vi "LOAD SELECTION MAIN CODE.vi"(8 "error in (no error)":errorcluster, 11 "main ref":T1) -> (0 "error out":errorcluster)   [LabVIEW 2025]
uses:
  controls/LAB-IQ UI Data.ctl
  <vilib>/addons/control/pid/pid.llb/PID Output Rate Limiter (DBL).vi
  <vilib>/addons/control/pid/NI_PID_pid.lvlib
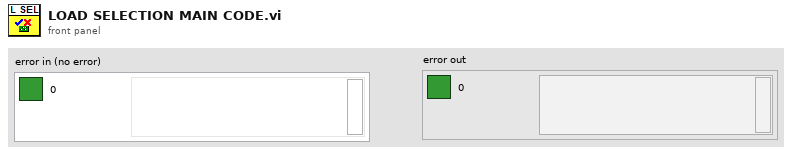
[diagram p1: front panel]
types:
  T1 = typedef "LAB-IQ UI Data.ctl" = cluster{"Main Home Screen":cluster{"GUI":refnum<vi>, "Platform Settings":refnum<vi>, "Configure":refnum<vi>, "Home":refnum<vi>, "EXIT":refnum<vi>, "service 2":refnum<vi>, "MainPage":refnum<vi>, "Analysis":refnum<vi>}, "Platform Settings":cluster{"mm/s  Surge":refnum<vi>, "Update Surge Speed":refnum<vi>, "Drive Error":refnum<vi>, "Disable Axis Jog Soft Limits":refnum<vi>, "mm/s  Sway":refnum<vi>, "Sway and Surge COM Status":refnum<vi>, "Heave COM Status":refnum<vi>, "Enable Platform":refnum<vi>, "Surge Forward Main":refnum<vi>, "Sway Right Main":refnum<vi>, "Sway Left Main":refnum<vi>, "Heave Down Main":refnum<vi>, "Heave Up main":refnum<vi>, "Update Sway Speed":refnum<vi>, "Update Heave Speed":refnum<vi>, "mm/s Heave":refnum<vi>, "mm/sec":refnum<vi>, "mm":refnum<vi>, "Surge Backward Main":refnum<vi>}, "Analysis Screen":cluster{"Analysis Home":refnum<vi>, "Surface Analysis":refnum<vi>, "Imaging":refnum<vi>, "Image Analysis":refnum<vi>, "Post Analysis":refnum<vi>}, "Config Screen":cluster{"Select Load Head":refnum<vi>, "Notes :":refnum<vi>, "FILE":refnum<vi>, "Sample ID :":refnum<vi>, "Operator ID :":refnum<vi>, "Operator Name :":refnum<vi>, "Auto":refnum<vi>}, "Motion Module":cluster{"zNL":refnum<vi>, "NL disp":refnum<vi>, "Rotary Tab":refnum<vi>, "Motion Direction:  3":refnum<vi>, "E.Velocity 2":refnum<vi>, "e.v/ssr 2":refnum<vi>, "Enter Fixed E.Velocity 2":refnum<vi>, "Enter Final SRR 2":refnum<vi>, "Enter initial SRR 2":refnum<vi>, "Enter Fixed SRR 2":refnum<vi>, "Enter the Final E.Velocity (m/s) 2":refnum<vi>, "Enter initial E.Velocity (m/s) 2":refnum<vi>, "Final Speed (RPM) 3":refnum<vi>, "Initial Speed (RPM) 2":refnum<vi>, "Enter the Final Velocity (m/s) 3":refnum<vi>, "Enter initial Velocity (m/s)  3":refnum<vi>, "Ramp Up 2":refnum<vi>, "TEST SELECTION":refnum<vi>, "SPEED SELECTION : ":refnum<vi>, "Angular Oscillation Set":refnum<vi>, "Traction":refnum<vi>, "Step Speed":refnum<vi>, "StepTable For Load-Speed":refnum<vi>, "StepTable For Speed":refnum<vi>, "Surge Forward MM":refnum<vi>, "Surge Backward MM":refnum<vi>, "M3 Image":refnum<vi>, "String 39":refnum<vi>, "Sway Left MM":refnum<vi>, "Sway Right MM":refnum<vi>, "Disable Axis Jog Soft Limits":refnum<vi>, "mm":refnum<vi>, "Heave Down MM":refnum<vi>, "Heave Up MM":refnum<vi>, "Wear Track Diameter (mm)":refnum<vi>, "Set WTD":refnum<vi>, "HomeScratch":refnum<vi>, "HomeRot":refnum<vi>, "PlaceModule":refnum<vi>, "Enter the Angle (Deg)":refnum<vi>, "Enter the Frequency (Hz)":refnum<vi>, "Motion Mode:":refnum<vi>, "LR Sway":refnum<vi>, "Rot Hor":refnum<vi>, "Scratch":refnum<vi>, "LR Cam":refnum<vi>, "MMBack":refnum<vi>, "MMNext":refnum<vi>, "Rot Ver":refnum<vi>, "Rotary Module Selection":refnum<vi>, "calculate rotary":refnum<vi>, "SPEED SELECTION : rotary":refnum<vi>, "Import 2":refnum<vi>, "Save 2":refnum<vi>, "File Path :  2":refnum<vi>, "String 45":refnum<vi>, "StepTable For Speed 3":refnum<vi>, "Enter the Speed(mm/sec)":refnum<vi>, "Enter the Speed(RPM)":refnum<vi>, "Enter Scratch Speed (mm/s):":refnum<vi>, "SwaySpeed Set":refnum<vi>, "Scartch Offset":refnum<vi>, "Motion type:":refnum<vi>, "HomeScratch 2":refnum<vi>, "Enter Scratch length (mm):":refnum<vi>, "Wear Track Diameter":refnum<vi>, "Rotary Speed Exced":refnum<vi>, "Scratch Mode":refnum<vi>, "No of Scratch":refnum<vi>}, "Environmental control":cluster{"Humidity  Status  3":refnum<vi>, "Low Temp  Status  2":refnum<vi>, "TK4 status 2":refnum<vi>, "Stage Temperature":refnum<vi>, "Sample Temperature":refnum<vi>, "Humidity (Amb)":refnum<vi>, "Clear List":refnum<vi>, "Add to list":refnum<vi>, "Wear":refnum<vi>, "Vibration":refnum<vi>, "Humidity (Chamber)":refnum<vi>, "Temperature (Chamber)":refnum<vi>, "ECR ":refnum<vi>, "Temperature (Amb)":refnum<vi>, "Microphone":refnum<vi>, "Acoustic Emission 3":refnum<vi>, "SNext":refnum<vi>, "APBack":refnum<vi>, "Enter the Temperature (°C):":refnum<vi>, "Enter the Stage \nTemperature (°C):":refnum<vi>, "Enter the Humidity (%Rh):":refnum<vi>, "Low Temp":refnum<vi>, "High Temp":refnum<vi>, "Humidity":refnum<vi>, "Sensors Picked":refnum<vi>}, "About Screen":cluster{"Password":refnum<vi>, "Home Service":refnum<vi>, "Advanced Setting":refnum<vi>, "About Tab":refnum<vi>, "ECR Port:":refnum<vi>, "Ramp Port:":refnum<vi>, "Installation/Replacement completed":refnum<vi>, "Loahead":refnum<vi>, "Heave and Surge COM Port:":refnum<vi>, "Sway COM Port:":refnum<vi>, "Temp Modbus:":refnum<vi>, "Humidity Port:":refnum<vi>, "Edit Gain Constants":refnum<vi>, "Save Gain Constants":refnum<vi>}, "Main Screen":cluster{"Main Screen Tab":refnum<vi>, "Angle and Frequency":refnum<vi>, "Stroke (mm)":refnum<vi>, "Angle (Deg)":refnum<vi>, "Main Speed Tab":refnum<vi>, "MTM MOTOR DISPLAY":refnum<vi>, "Disc Speed (m/sec)":refnum<vi>, "Ball Speed (m/sec)":refnum<vi>, "Disc Speed (RPM)":refnum<vi>, "Ball Speed (RPM)":refnum<vi>, "SPEED TAB":refnum<vi>, "Speed (m/sec)":refnum<vi>, "Set Speed (m/sec)":refnum<vi>, "Speed (RPM)":refnum<vi>, "Set Speed":refnum<vi>, "Time Tab":refnum<vi>, "Time ( HH:MM:SS ) 2":refnum<vi>, "Test Duration":refnum<vi>, "Test Duration 4":refnum<vi>, "TEST CYCLE":refnum<vi>, "TOTAL CYCLES":refnum<vi>, "Set Load (N)":refnum<vi>, "Temp Tabs":refnum<vi>, "Heater":refnum<vi>, "TK4 status":refnum<vi>, "ChamberTemp":refnum<vi>, "SetTmp":refnum<vi>, "Controller  Status":refnum<vi>, "ChamberTemp 2":refnum<vi>, "SetTmp 2":refnum<vi>, "Controller  Status 2":refnum<vi>, "ChamberTemp 3":refnum<vi>, "SetTmp 3":refnum<vi>, "Cooling":refnum<vi>, "Load Communication":refnum<vi>, "Ambient \nTemperature":refnum<vi>, "HumCOMStatus":refnum<vi>, "Ambient\n Humidity":refnum<vi>, "Freq (Hz)":refnum<vi>, "Load En":refnum<vi>, "NLt":refnum<vi>, "zNL 2":refnum<vi>, "Humidity On":refnum<vi>, "humidity disp":refnum<vi>, "Set Humidity":refnum<vi>, "NL disp 2":refnum<vi>, "Humidity On 2":refnum<vi>, "humidity disp 2":refnum<vi>, "Set Humidity 2":refnum<vi>, "NL disp 3":refnum<vi>, "AppLoadSeq scratch":refnum<vi>, "Stop Scratch":refnum<vi>, "ClrLog":refnum<vi>, "Trip Log":refnum<vi>, "STOP":refnum<vi>, "Start Test":refnum<vi>, "Test status":refnum<vi>, "AR Led":refnum<vi>, "Data":refnum<vi>, "Health":refnum<vi>, "Sway COM Status":refnum<vi>, "Heave COM Status":refnum<vi>, "Grp Tab":refnum<vi>, "Sub Graph":refnum<vi>, "SD (mm)":refnum<vi>, "Siliding distance Reset Graph":refnum<vi>, "SDGp":refnum<vi>, "Humidity Reset Graph":refnum<vi>, "HumrGp":refnum<vi>, "Acoustic Emission (mV)":refnum<vi>, "Aqucostic Reset Graph":refnum<vi>, "gACQUOS":refnum<vi>, "ECR RESET":refnum<vi>, "ECR":refnum<vi>, "Temperature Reset":refnum<vi>, "Acoustic Emission (mV) 2":refnum<vi>, "Aqucostic Reset Graph 2":refnum<vi>, "gACQUOS 2":refnum<vi>, "ECR RESET 2":refnum<vi>, "ECR 2":refnum<vi>, "Temperature Reset 2":refnum<vi>, "Temperature (deg c)":refnum<vi>, "Speed Reset Graph":refnum<vi>, "Speed Tab":refnum<vi>, "MTM DISC  SPEED":refnum<vi>, "MTM BALL SPEED":refnum<vi>, "speed mm/sec":refnum<vi>, "Hymidity":refnum<vi>, "Humidity Disable trip":refnum<vi>, "CoF Trip  2":refnum<vi>, "Depth Trip":refnum<vi>, "Weart Deapth":refnum<vi>, "Depth Reset Graph":refnum<vi>, "Weart":refnum<vi>, "Depthz":refnum<vi>, "Depth (µm)":refnum<vi>, "WearGp":refnum<vi>, "NL Trip 2":refnum<vi>, "Load pid":refnum<vi>, "Load Disable Trip":refnum<vi>, "Load Reset Graph":refnum<vi>, "NL Display 4":refnum<vi>, "Main Chart 3":refnum<vi>, "BACK":refnum<vi>, "Depth Trip 2":refnum<vi>, "COF TRIP ":refnum<vi>, "Friction Force (N)":refnum<vi>, "FF Reset Graph":refnum<vi>, "FF Disable Trip":refnum<vi>, "FF TRIP":refnum<vi>, "COF Disable Trip":refnum<vi>, "COF Reset Graph":refnum<vi>, "Start Test Temp":refnum<vi>, "zFF":refnum<vi>, "Friction Force (N) Graph":refnum<vi>, "Coefficient of Friction":refnum<vi>, "Scratch Start Test":refnum<vi>, "FF Tab":refnum<vi>, "Cyclic Friction Force (N)":refnum<vi>, "CZ FF":refnum<vi>, "Cyclic Friction Force (N) Graph":refnum<vi>, "Cyclic Coefficient of Friction":refnum<vi>, "Cyclic FF TRIP":refnum<vi>, "Cyclic FF Disable Trip":refnum<vi>, "cyclic COF Disable Trip":refnum<vi>, "cyclic COF TRIP":refnum<vi>, "cyclic COF Reset Graph":refnum<vi>, "Cyclic FF Reset Graph":refnum<vi>, "Test Trip":refnum<vi>, "Multi Scratch Pass":refnum<vi>}, "Loading":cluster{"Indentation":refnum<vi>, "Reference Sample":refnum<vi>, "Load Cell Communication Slide":refnum<vi>, "com 3":refnum<vi>, "com":refnum<vi>, "DecaForce COM Status":refnum<vi>, "Update":refnum<vi>, "Clear 3":refnum<vi>, "seq":refnum<vi>, "Stribeck table":refnum<vi>, "Stribeck Table  For loading":refnum<vi>, "Loading Mode":refnum<vi>, "Enter the Final Load (N)":refnum<vi>, "Enter the CoF Trip":refnum<vi>, "Enter the Friction Force Trip":refnum<vi>, "Enter the Normal load Trip":refnum<vi>, "Enter the Load  (N)":refnum<vi>, "KiloForce":refnum<vi>, "DecaForce ":refnum<vi>, "MicroForce":refnum<vi>, "LHBack":refnum<vi>, "LHNext":refnum<vi>, "Enter the Loading Rate (N/min)":refnum<vi>, "Message":refnum<vi>, "Warning 2":refnum<vi>, "SSP 0.75":refnum<vi>, "SSP 0.5":refnum<vi>, "SSP 0.3":refnum<vi>, "Warning":refnum<vi>, "gui GIF":refnum<vi>, "Communication is established":refnum<vi>, "AppLoad 4":refnum<vi>, "Multipoint":refnum<vi>, "Load Selection":refnum<vi>}, "PID":cluster{"Ramp MulFac":refnum<vi>, "pulses LoadDiffRamp(2..10)":refnum<vi>, "PulseControlRamp(diff<=3N)":refnum<vi>, "SetLoadDeadband(%) Load(0-10N)":refnum<vi>, "PID gains out delay (microForce)":refnum<vi>, "Ramp":refnum<vi>, "Gain 2":refnum<vi>, "pulses LoadDiff(2..10)":refnum<vi>, "pulses LoadDiff(11..50)":refnum<vi>, "PulseControl(diff<=3N)":refnum<vi>, "SetLoadDeadband(%)  2":refnum<vi>, "Dummy Run":refnum<vi>, "Vertical load (N)":refnum<vi>, "AutoTune":refnum<vi>, "Offset 3 ":refnum<vi>, "apply load":refnum<vi>, "Offset  3":refnum<vi>, "apply load 2":refnum<vi>, "Enter ByPass Load":refnum<vi>, "reinit 3":refnum<vi>, "output range delay":refnum<vi>, "PID gains out delay":refnum<vi>, "Bypass Load":refnum<vi>, "pulsesSent":refnum<vi>, "pulses ":refnum<vi>, "actpid":refnum<vi>, "gFF Rot":refnum<vi>, "pulses LoadDiff(21..1000)":refnum<vi>, "Delay":refnum<vi>, "deadband":refnum<vi>}, "Config Parameters":cluster{"Tab Control 3":refnum<vi>, "Tab Control 19":refnum<vi>, "SAMPLES":refnum<vi>, "Re-initilaize":refnum<vi>, "Filter ON/OFF":refnum<vi>, "TracHomeSurgeOffsetCounts 10MM":refnum<vi>, "TracHomeSwayOffsetCounts 10MM":refnum<vi>, "Acoustic Emission:":refnum<vi>, "Apply Filter (FF)":refnum<vi>, "Filter% 2":refnum<vi>, "Apply Filter (Load)":refnum<vi>, "Filter% ":refnum<vi>, "Sway distance (mm)":refnum<vi>, "Surge distance (mm)":refnum<vi>, "DataSavingLoopDelay(ms)":refnum<vi>, "SAVE 2":refnum<vi>, "Enter Distance":refnum<vi>, "Sway Counts:":refnum<vi>, "Distance (mm): 3":refnum<vi>, "Surge Counts:":refnum<vi>, "Distance (mm): 2":refnum<vi>, "Distance (mm):":refnum<vi>, "Heave Counts:":refnum<vi>, "LRMHomeSurgeOffsetCounts":refnum<vi>, "LRMHomeSwayOffsetCounts":refnum<vi>, "TracHomeSurgeOffsetCounts 20MM":refnum<vi>, "TracHomeSwayOffsetCounts 20MM":refnum<vi>, "RotHomeSwayOffsetCounts":refnum<vi>, "RotHomeSurgeOffsetCounts":refnum<vi>, "Heave distance":refnum<vi>, "Zmm":refnum<vi>, "Heave Pulses/mm":refnum<vi>, "Surge Pulses/mm":refnum<vi>, "Sway Pulses/mm":refnum<vi>, "Heave Pitch":refnum<vi>, "Surge Pitch":refnum<vi>, "Sway Pitch":refnum<vi>, "Heave PPR":refnum<vi>, "Surge PPR":refnum<vi>, "Sway PPR":refnum<vi>, "Tab Control 5":refnum<vi>, "Tab Control 14":refnum<vi>, "Tab Control 26":refnum<vi>, "AE":refnum<vi>, "Heave Loop Delay":refnum<vi>, "Heave PID Speed":refnum<vi>, "Surge Jog Speed":refnum<vi>, "Heave Jog Speed":refnum<vi>, "Sway Loop Delay":refnum<vi>, "Sway PID Speed":refnum<vi>, "Sway Jog Speed":refnum<vi>}, "Loading Com Port":cluster{"ClearAll":refnum<vi>, "Mz(Nm)":refnum<vi>, "My(Nm)":refnum<vi>, "Mx(Nm)":refnum<vi>, "Save Dwell":refnum<vi>, "Mx ":refnum<vi>, "My ":refnum<vi>, "Mz":refnum<vi>, "Fx(N)":refnum<vi>, "Fy(N)":refnum<vi>, "Fz(N)":refnum<vi>, "ZeroAll":refnum<vi>, "Acq Delay (ms)":refnum<vi>, "Burst Delay (ms)":refnum<vi>, "model":refnum<vi>, "SN":refnum<vi>, "FFx(N)":refnum<vi>, "Sensor IP":refnum<vi>, "Port":refnum<vi>, "FFy(N)":refnum<vi>, "Load(N)":refnum<vi>, "delete Handle":refnum<vi>, "Create Handle":refnum<vi>, "ft_data":refnum<vi>, "ft_range":refnum<vi>, "ft_data 2":refnum<vi>, "stop 6":refnum<vi>, "running_flag":refnum<vi>, "ft_udp_handle":refnum<vi>, "get-data-return":refnum<vi>, "get-range-return":refnum<vi>, "zero-return":refnum<vi>, "filter-return":refnum<vi>, "initial-return":refnum<vi>, "deleteHandle-result":refnum<vi>, "Load Cell Temp":refnum<vi>}, "Heave AND Surge":cluster{"SURGE POSE":refnum<vi>, "error out Read":refnum<vi>, "HEAVE POSE":refnum<vi>, "State":refnum<vi>, "Homed":refnum<vi>, "Sequence ID":refnum<vi>, "error out Write":refnum<vi>, "faultCode":refnum<vi>, "Ack ID":refnum<vi>, "SPEED":refnum<vi>, "Distance":refnum<vi>, "Mode Command":refnum<vi>, "Heave and Surge Read":refnum<vi>, "Read Heave Temp":refnum<vi>, "Spare 15":refnum<vi>, "Spare 14":refnum<vi>, "Spare 13":refnum<vi>, "Spare 12":refnum<vi>, "Spare 11":refnum<vi>, "Spare 10":refnum<vi>, "Spare 9":refnum<vi>, "Spare 8":refnum<vi>, "Spare 7":refnum<vi>, "Spare 6":refnum<vi>, "Spare 5":refnum<vi>, "Spare 4":refnum<vi>, "Spare 2":refnum<vi>, "Spare 1":refnum<vi>, "Node Id":refnum<vi>, "Spare 3":refnum<vi>, "SPARE 4":refnum<vi>, "SPARE 3":refnum<vi>, "SPARE 2":refnum<vi>, "SPARE 1":refnum<vi>, "fwMajor":refnum<vi>, "fwMinor":refnum<vi>, "Manual Write":refnum<vi>, "Heave and Surge Write":refnum<vi>}, "New PID LOGIC":cluster{"Fine Tune Zone":refnum<vi>, "PID SDelay":refnum<vi>, "Max_pos_limit":refnum<vi>, "Min_pos_limit":refnum<vi>, "i_limit":refnum<vi>, "pct_scale":refnum<vi>, "Deadband":refnum<vi>, "Kd":refnum<vi>, "Ki":refnum<vi>, "Kp":refnum<vi>, "Current Position":refnum<vi>, "Set Load":refnum<vi>, "Current Load":refnum<vi>, "Pulse delta":refnum<vi>, "Init Step":refnum<vi>, "Max Step Linit":refnum<vi>}, "SWAY ":cluster{"fwMajor":refnum<vi>, "Homed":refnum<vi>, "Rotary POSE":refnum<vi>, "State":refnum<vi>, "SWAY POSE":refnum<vi>, "Ack ID":refnum<vi>, "faultCode":refnum<vi>, "Node Id":refnum<vi>, "fwMinor":refnum<vi>, "Spare 6":refnum<vi>, "Spare 5":refnum<vi>, "Spare 4":refnum<vi>, "Spare 3":refnum<vi>, "Spare 2":refnum<vi>, "Spare 1":refnum<vi>, "Spare 7":refnum<vi>, "SPARE  5":refnum<vi>, "error out Write  SWAY ":refnum<vi>, "error out Read SWAY ":refnum<vi>, "Manual Write SWAY ":refnum<vi>, "SWAY WRITE":refnum<vi>, "SPARE  4":refnum<vi>, "SPARE  3":refnum<vi>, "SPARE 2":refnum<vi>, "SPARE 1":refnum<vi>, "Spare 15":refnum<vi>, "Spare 14":refnum<vi>, "Spare 13":refnum<vi>, "Spare 12":refnum<vi>, "Spare 11":refnum<vi>, "Spare 9":refnum<vi>, "Spare 8":refnum<vi>, "SPEED":refnum<vi>, "Distance":refnum<vi>, "Mode Command":refnum<vi>, "Sequence ID":refnum<vi>, "SWAY READ":refnum<vi>, "Spare 10":refnum<vi>, "Read SWAY Temp":refnum<vi>}, "Analysis Screen":cluster{"Analysis Home":refnum<vi>, "Refresh 2":refnum<vi>, "MEAN 4":refnum<vi>, "SD 4":refnum<vi>, "VARIANCE 4":refnum<vi>, "MEAN  3":refnum<vi>, "SD  3":refnum<vi>, "VARIANCE  3":refnum<vi>, "MEAN 2":refnum<vi>, "SD  2":refnum<vi>, "VARIANCE 2":refnum<vi>, "MEAN":refnum<vi>, "SD":refnum<vi>, "VARIANCE":refnum<vi>, "File 4 Discription":refnum<vi>, "OPEN 4":refnum<vi>, "File Name 4":refnum<vi>, "OPEN 3":refnum<vi>, "File 3 Discription":refnum<vi>, "File Name 3":refnum<vi>, "Y-AXIS":refnum<vi>, "X-AXIS":refnum<vi>, "XY Graph":refnum<vi>, "File Name 2":refnum<vi>, "File Name 1":refnum<vi>, "OPEN 2":refnum<vi>, "OPEN 1":refnum<vi>, "File 1 Discription ":refnum<vi>, "File 2 Discription":refnum<vi>}}
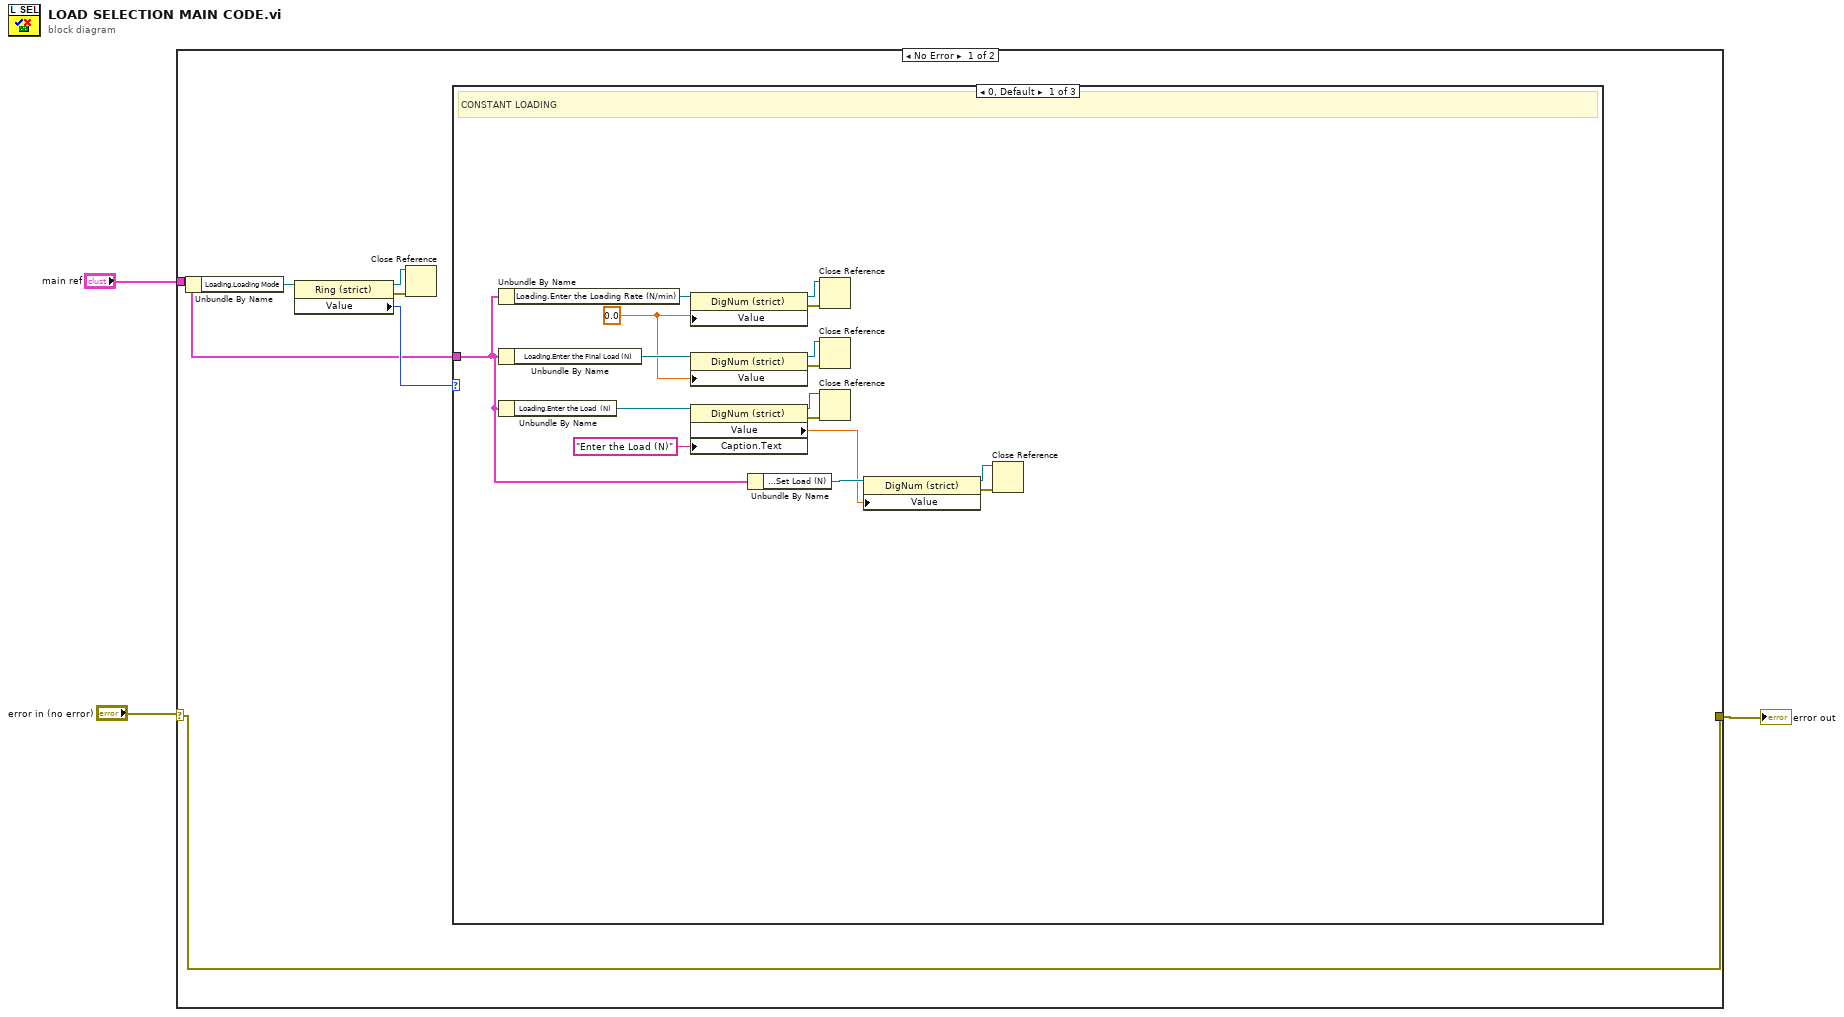
[diagram p0: block diagram]
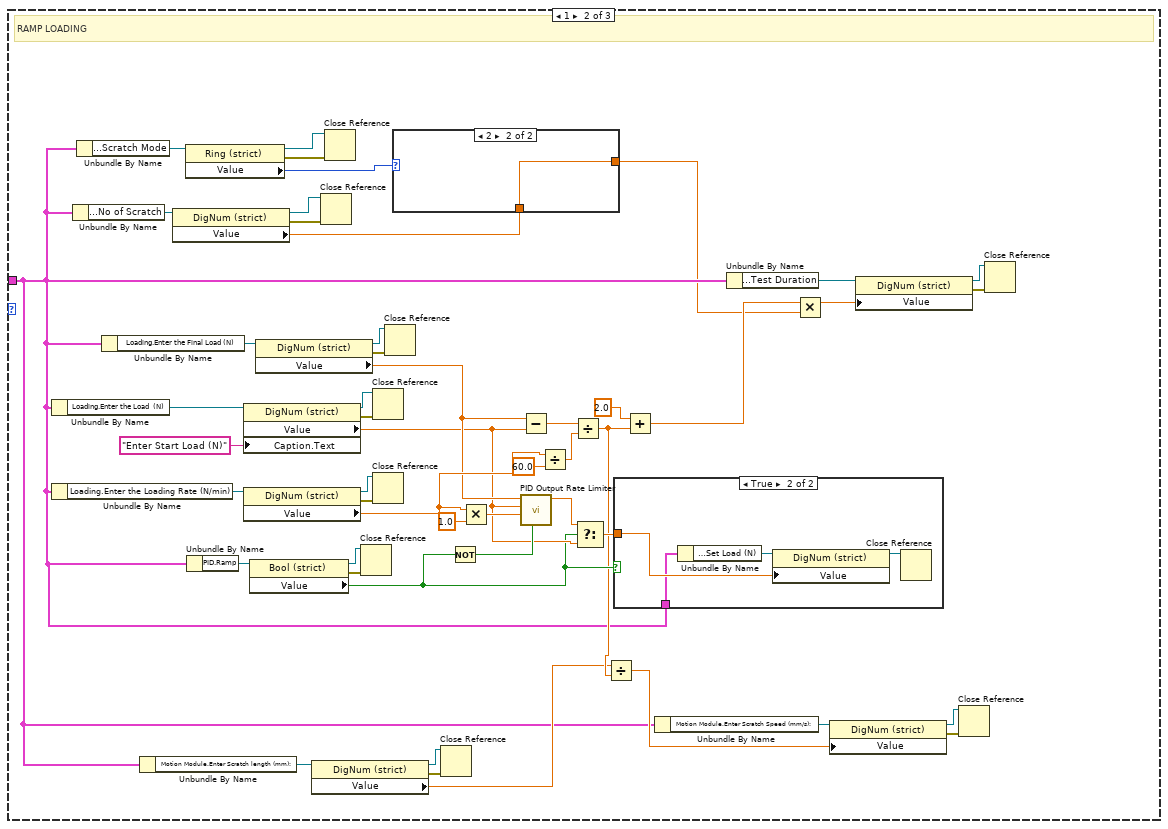
[diagram p2: hidden frame]
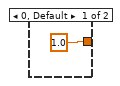
[diagram p3: hidden frame]
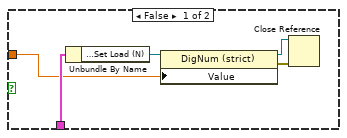
[diagram p4: hidden frame]
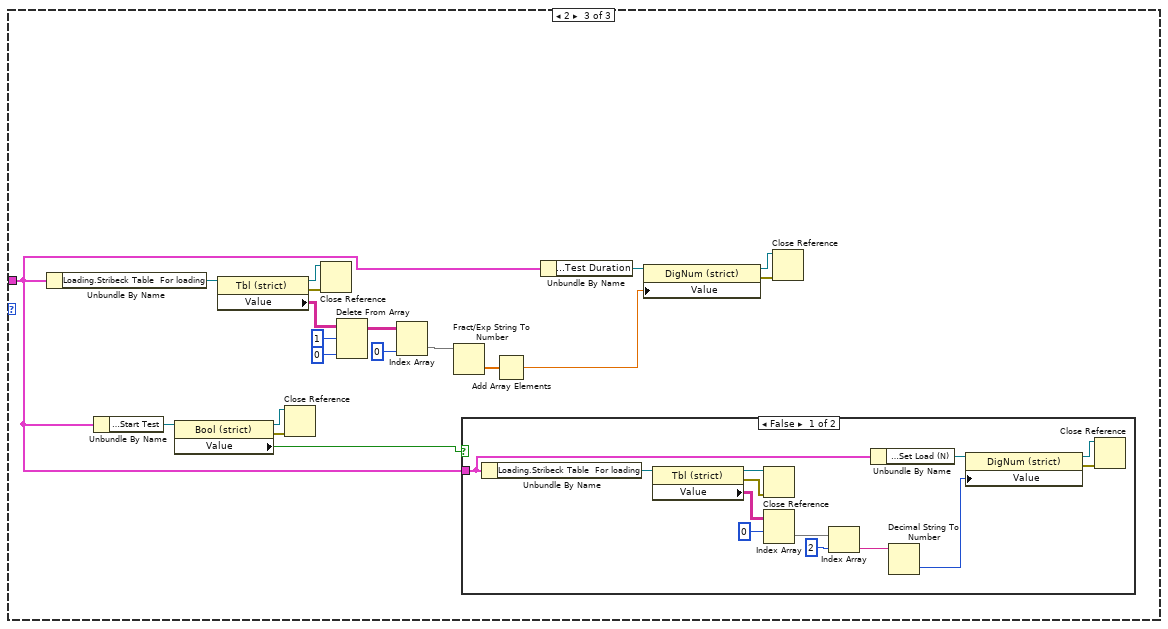
[diagram p5: hidden frame]
diagram:
  n1 = case shown="No Error" "error in (no error)" {
    selector: "error in (no error)" -> [w4 _]
    tunnel: "main ref" -> [w5 _]
    tunnel: [w4 _] -> w1
    frame No Error {
      n2 = Unbundle By Name(w5) -> ("Loading.Loading Mode"=w9:refnum<vi>)
      n3 = property class="Ring (strict)"(reference=w9) -> (reference out=w7:refnum<vi>, error out=w8:errorcluster, "Value"=w6:u16)  [unwired: 1 in]
      n4 = Close Reference(reference=w7, error in (no error)=w8) -> ()  [unwired: 1 out]
      n5 = case shown="0, Default" w6 {
        tunnel: w5 -> [w12 w28 w89]
        frame 0, Default {
          w16 = 0.0 ("Value")
          # "CONSTANT LOADING"
          n6 = Unbundle By Name(w12) -> ("Loading.Enter the Loading Rate (N/min)"=w19:refnum<vi>)
          n7 = Unbundle By Name(w12) -> ("Loading.Enter the Final Load (N)"=w23:refnum<vi>)
          n8 = Unbundle By Name(w12) -> ("Loading.Enter the Load  (N)"=w22:refnum<vi>)
          n9 = property class="DigNum (strict)"(reference=w19, "Value"=w16) -> (reference out=w17:refnum<vi>, error out=w18:errorcluster)  [unwired: 1 in]
          n10 = property class="DigNum (strict)"(reference=w23, "Value"=w16) -> (reference out=w25:refnum<vi>, error out=w24:errorcluster)  [unwired: 1 in]
          n11 = property class="DigNum (strict)"(reference=w22, "Caption.Text"="Enter the Load (N)") -> (reference out=w20:refnum<vi>, error out=w21:errorcluster, "Value"=w11:dbl)  [unwired: 1 in]
          n12 = Unbundle By Name(w12) -> ("Main Screen.Set Load (N)"=w13:refnum<vi>)
          n13 = Close Reference(reference=w17, error in (no error)=w18) -> ()  [unwired: 1 out]
          n14 = Close Reference(reference=w25, error in (no error)=w24) -> ()  [unwired: 1 out]
          n15 = Close Reference(reference=w20, error in (no error)=w21) -> ()  [unwired: 1 out]
          n16 = property class="DigNum (strict)"(reference=w13, "Value"=w11) -> (reference out=w15:refnum<vi>, error out=w14:errorcluster)  [unwired: 1 in]
          n17 = Close Reference(reference=w15, error in (no error)=w14) -> ()  [unwired: 1 out]
        }
        frame 1 {
          # "RAMP LOADING"
          n18 = Unbundle By Name(w28) -> ("Loading.Enter the Load  (N)"=w72:refnum<vi>)
          n19 = Unbundle By Name(w28) -> ("Loading.Enter the Loading Rate (N/min)"=w69:refnum<vi>)
          n20 = Unbundle By Name(w28) -> ("Motion Module.No of Scratch"=w31:refnum<vi>)
          n21 = Unbundle By Name(w28) -> ("Motion Module.Scratch Mode"=w35:refnum<vi>)
          n22 = Unbundle By Name(w28) -> ("Loading.Enter the Final Load (N)"=w73:refnum<vi>)
          n23 = Unbundle By Name(w28) -> ("Motion Module.Enter Scratch length (mm):"=w42:refnum<vi>)
          n24 = property class="DigNum (strict)"(reference=w31) -> (reference out=w30:refnum<vi>, error out=w32:errorcluster, "Value"=w29:dbl)  [unwired: 1 in]
          n25 = property class="Ring (strict)"(reference=w35) -> (reference out=w36:refnum<vi>, error out=w34:errorcluster, "Value"=w33:u16)  [unwired: 1 in]
          n26 = Unbundle By Name(w28) -> ("PID.Ramp"=w52:refnum<vi>)
          n27 = property class="DigNum (strict)"(reference=w72, "Caption.Text"="Enter Start Load (N)") -> (reference out=w70:refnum<vi>, error out=w71:errorcluster, "Value"=w56:dbl)  [unwired: 1 in]
          n28 = property class="DigNum (strict)"(reference=w69) -> (reference out=w55:refnum<vi>, error out=w68:errorcluster, "Value"=w58:dbl)  [unwired: 1 in]
          n29 = property class="Bool (strict)"(reference=w52) -> (reference out=w54:refnum<vi>, error out=w53:errorcluster, "Value"=w51:bool)  [unwired: 1 in]
          n30 = property class="DigNum (strict)"(reference=w73) -> (reference out=w75:refnum<vi>, error out=w74:errorcluster, "Value"=w57:dbl)  [unwired: 1 in]
          n31 = property class="DigNum (strict)"(reference=w42) -> (reference out=w44:refnum<vi>, error out=w43:errorcluster, "Value"=w39:dbl)  [unwired: 1 in]
          n32 = Close Reference(reference=w30, error in (no error)=w32) -> ()  [unwired: 1 out]
          n33 = Close Reference(reference=w36, error in (no error)=w34) -> ()  [unwired: 1 out]
          n34 = Close Reference(reference=w54, error in (no error)=w53) -> ()  [unwired: 1 out]
          n35 = Close Reference(reference=w70, error in (no error)=w71) -> ()  [unwired: 1 out]
          n36 = Close Reference(reference=w55, error in (no error)=w68) -> ()  [unwired: 1 out]
          n37 = Close Reference(reference=w75, error in (no error)=w74) -> ()  [unwired: 1 out]
          n38 = case shown="2" w33 {
            tunnel: [1.0 w77] -> w26
            tunnel: w29 -> [_ w77]
            frame 0, Default {
            }
            frame 2 {
            }
          }
          n39 = Close Reference(reference=w44, error in (no error)=w43) -> ()  [unwired: 1 out]
          n40 = Not(x=w51) -> (.not. x?=w64:bool)
          n41 = Multiply(x=w58, y=1.0) -> (x*y=w61:dbl)
          n42 = Subtract(x=w57, y=w56) -> (x-y=w65:dbl)
          n43 = call-poly <vilib>:"PID Output Rate Limiter.vi"("reinitialize? (F)"=w64, "output rate (EGU/min)"=w61, "initial output"=w56, "input (controller output)"=w57) -> ("output"=w62:dbl)  [unwired: 4 in, 1 out]
          n44 = Divide(x=w58, y=60.0) -> (x/y=w66:dbl)
          n45 = Divide(x=w65, y=w66) -> (x/y=w40:dbl)
          n46 = Select(t=w62, s=w51, f=w56) -> (s? t:f=w63:dbl)
          n47 = Divide(x=w39, y=w40) -> (x/y=w41:dbl)
          n48 = case shown="True" w51 {
            tunnel: w63 -> [w78 w84]
            tunnel: w28 -> [w80 w83]
            frame False {
              n49 = Unbundle By Name(w80) -> ("Main Screen.Set Load (N)"=w81:refnum<vi>)
              n50 = property class="DigNum (strict)"(reference=w81, "Value"=w78) -> (reference out=w82:refnum<vi>, error out=w79:errorcluster)  [unwired: 1 in]
              n51 = Close Reference(reference=w82, error in (no error)=w79) -> ()  [unwired: 1 out]
            }
            frame True {
              n52 = Unbundle By Name(w83) -> ("Main Screen.Set Load (N)"=w85:refnum<vi>)
              n53 = property class="DigNum (strict)"(reference=w85, "Value"=w84) -> (reference out=w86:refnum<vi>)  [unwired: 1 in, 1 out]
              n54 = Close Reference(reference=w86) -> ()  [unwired: 1 in, 1 out]
            }
          }
          n55 = Add(x=2.0, y=w40) -> (x+y=w38:dbl)
          n56 = Unbundle By Name(w28) -> ("Motion Module.Enter Scratch Speed (mm/s):"=w47:refnum<vi>)
          n57 = Unbundle By Name(w28) -> ("Main Screen.Test Duration"=w50:refnum<vi>)
          n58 = Multiply(x=w38, y=w26) -> (x*y=w27:dbl)
          n59 = property class="DigNum (strict)"(reference=w47, "Value"=w41) -> (reference out=w45:refnum<vi>, error out=w46:errorcluster)  [unwired: 1 in]
          n60 = property class="DigNum (strict)"(reference=w50, "Value"=w27) -> (reference out=w48:refnum<vi>, error out=w49:errorcluster)  [unwired: 1 in]
          n61 = Close Reference(reference=w45, error in (no error)=w46) -> ()  [unwired: 1 out]
          n62 = Close Reference(reference=w48, error in (no error)=w49) -> ()  [unwired: 1 out]
        }
        frame 2 {
          n63 = Unbundle By Name(w89) -> ("Loading.Stribeck Table  For loading"=w105:refnum<vi>)
          n64 = Unbundle By Name(w89) -> ("Main Screen.Start Test"=w91:refnum<vi>)
          n65 = property class="Bool (strict)"(reference=w91) -> (reference out=w88:refnum<vi>, error out=w90:errorcluster, "Value"=w87:bool)  [unwired: 1 in]
          n66 = property class="Tbl (strict)"(reference=w105) -> (reference out=w103:refnum<vi>, error out=w104:errorcluster, "Value"=w102:string[][])  [unwired: 1 in]
          n67 = Close Reference(reference=w88, error in (no error)=w90) -> ()  [unwired: 1 out]
          n68 = Close Reference(reference=w103, error in (no error)=w104) -> ()  [unwired: 1 out]
          n69 = Delete From Array(array=w102, length=1, index (col)=0 ("disabled index (col)")) -> (array with subset deleted=w99:string[][])  [unwired: 1 in, 1 out]
          n70 = Index Array(array=w99, index (col)=0 ("disabled index (col)")) -> (element=w97:string[])  [unwired: 1 in]
          n71 = Fract/Exp String To Number(string=w97) -> (number=w96:dbl[])  [unwired: 3 in, 1 out]
          n72 = case shown="False" w87 {
            tunnel: w89 -> [w109 _]
            frame False {
              n73 = Unbundle By Name(w109) -> ("Loading.Stribeck Table  For loading"=w116:refnum<vi>)
              n74 = property class="Tbl (strict)"(reference=w116) -> (reference out=w114:refnum<vi>, error out=w115:errorcluster, "Value"=w113:string[][])  [unwired: 1 in]
              n75 = Close Reference(reference=w114, error in (no error)=w115) -> ()  [unwired: 1 out]
              n76 = Index Array(array=w113, index (row)=0) -> (element=w118:string[])  [unwired: 1 in]
              n77 = Index Array(array=w118, index=2) -> (element=w108:string)
              n78 = Unbundle By Name(w109) -> ("Main Screen.Set Load (N)"=w112:refnum<vi>)
              n79 = Decimal String To Number(string=w108) -> (number=w107:i32)  [unwired: 2 in, 1 out]
              n80 = property class="DigNum (strict)"(reference=w112, "Value"=w107) -> (reference out=w110:refnum<vi>, error out=w111:errorcluster)  [unwired: 1 in]
              n81 = Close Reference(reference=w110, error in (no error)=w111) -> ()  [unwired: 1 out]
            }
            frame True {
            }
          }
          n82 = Add Array Elements(numeric array=w96) -> (sum=w92:dbl)
          n83 = Unbundle By Name(w89) -> ("Main Screen.Test Duration"=w93:refnum<vi>)
          n84 = property class="DigNum (strict)"(reference=w93, "Value"=w92) -> (reference out=w95:refnum<vi>, error out=w94:errorcluster)  [unwired: 1 in]
          n85 = Close Reference(reference=w95, error in (no error)=w94) -> ()  [unwired: 1 out]
        }
      }
    }
    frame Error {
    }
  }
  "error out" <- w1
